vi "Debug_Convert_Data_to_String.vi"(8 "error in (no error)":errorcluster, 11 "AB_Application in":refnum<class "AB_Application.lvclass">) -> (0 "error out":errorcluster, 2 "classData":string, 3 "AB_Application out":refnum<class "AB_Application.lvclass">)   [LabVIEW 2020, in "AB_Application.lvclass"]
uses:
  <vilib>/AppBuilder/AB_Classes/Application/AB_Application.lvclass
  <vilib>/AppBuilder/AB_Classes/Application/AB_Application.lvclass/AB_Application.ctl
  <vilib>/AppBuilder/AB_Classes/TargetFile/AB_Targetfile.lvclass
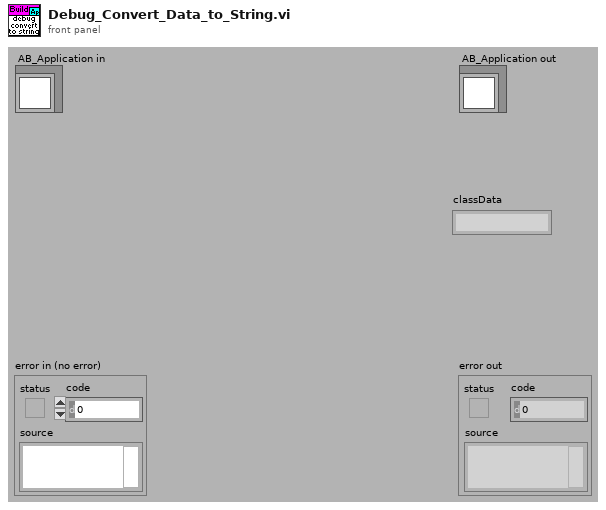
[diagram p1: front panel]
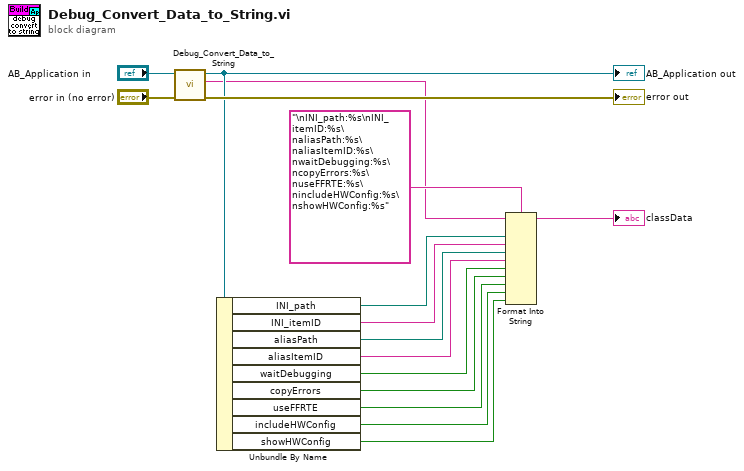
[diagram p0: block diagram]
diagram:
  n1 = call-parent "Debug_Convert_Data_to_String.vi"("error in (no error)"="error in (no error)", "AB_Targetfile in"="AB_Application in") -> ("error out"=→"error out":errorcluster, "classData"=w2:string, "AB_Targetfile out"=w12:refnum<class "AB_Application.lvclass">)  [unwired: 7 in]
  "AB_Application out" <- w12
  n2 = Unbundle By Name(w12) -> ("INI_path"=w11:path, "INI_itemID"=w10:string, "aliasPath"=w9:path, "aliasItemID"=w8:string, "waitDebugging"=w7:bool, "copyErrors"=w6:bool, "useFFRTE"=w5:bool, "includeHWConfig"=w4:bool, "showHWConfig"=w3:bool)
  n3 = Format Into String(format string="\nINI_path:%s\nINI_itemID:%s\naliasPath:%s\naliasItemID:%s\nwaitDebugging:%s\ncopyErrors:%s\nuseFFRTE:%s\nincludeHWConfig:%s\nshowHWConfig:%s", initial string=w2, w11, w10, w9, w8, w7, w6, w5, w4, w3) -> (resulting string=→"classData":string)  [unwired: 1 in, 1 out]
